vi "Tektronix_CollectWvfrm.vi"() -> ()   [LabVIEW 2018]
panel:
  in  "Collect Data":bool
  out "concatenated string":string
  out "Acquire Parameters":string
  out "output waveform 2":waveform(dbl)(graph)
  out "error out 2":errorcluster
  in  "End Point":i32
  in  "Start Point":i32
  in  "error in (no error)":errorcluster
  in  "Tektronix (0::20:)":refnum<visa-resource-name>
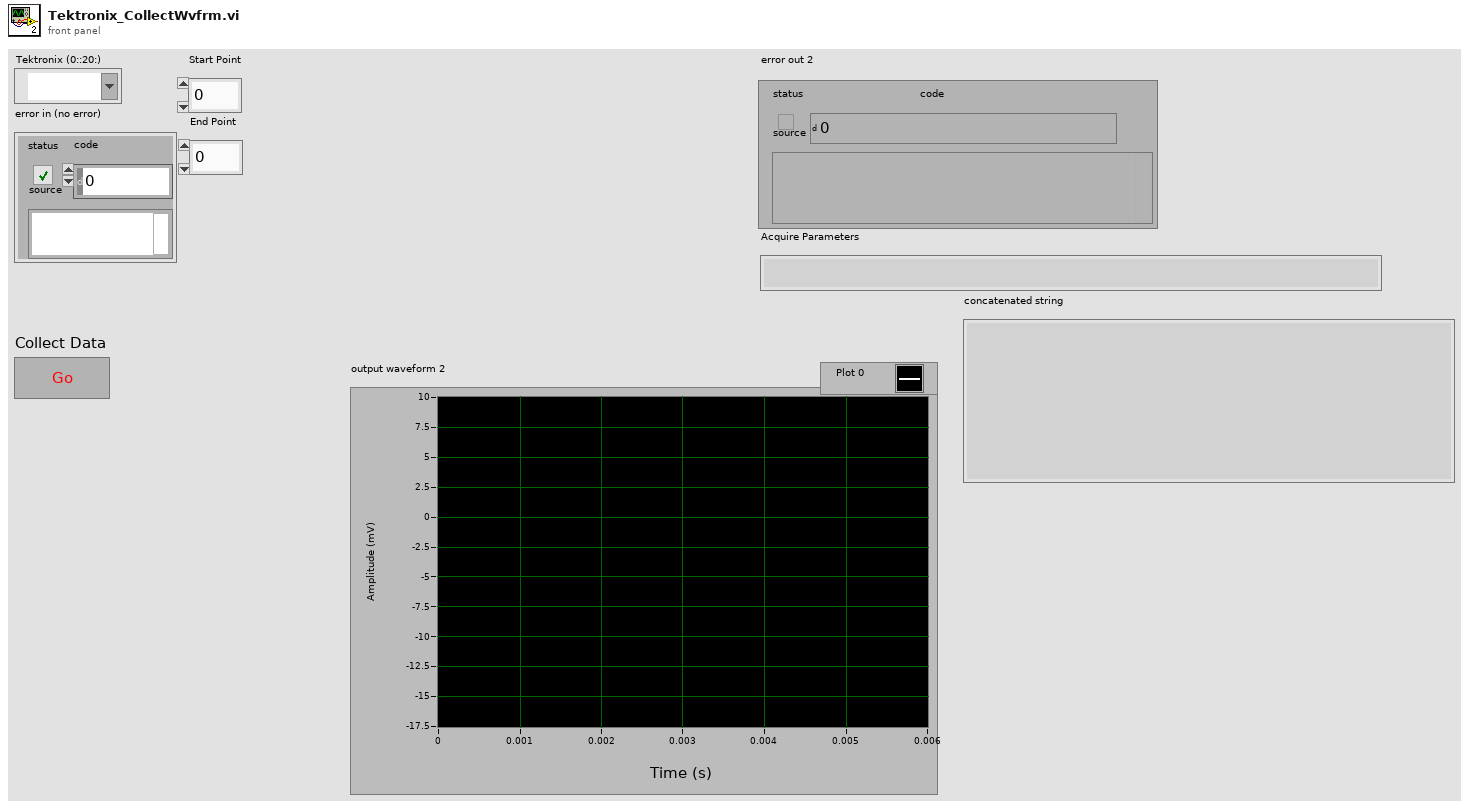
[diagram p1: front panel]
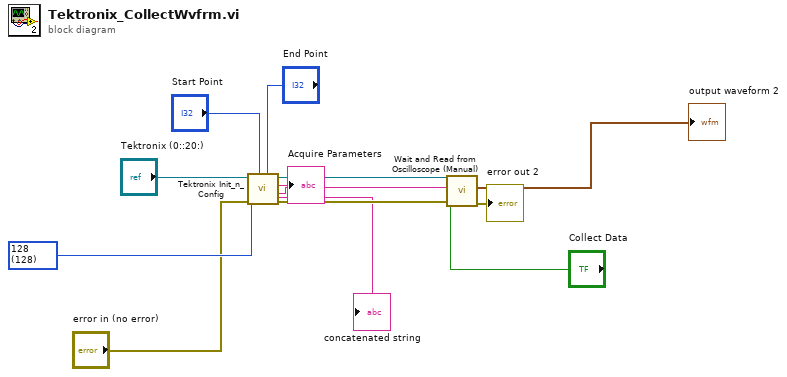
[diagram p0: block diagram]
diagram:
  w12 = u8 128 items=["128"=128, "64"=64, "16"=16, "4"=4] ("# Average")
  n1 = call "Tektronix Init_n_Config.vi"("End Point"="End Point", "Start Point"="Start Point", "error in (no error)"="error in (no error)", "# Average"=w12, "Tektronix (0::20:)"="Tektronix (0::20:)") -> ("error out"=w6:errorcluster, "Waveform Parameters"=w7:string, "Acquire Parameters"=→"Acquire Parameters":string, "VISA resource name out"=w8:refnum<visa-resource-name>, "concatenated string"=→"concatenated string":string)  [unwired: 2 in]
  n2 = call "Wait and Read from Oscilloscope (Manual).vi"("error in (no error)"=w6, "Collect Data"="Collect Data", "data format"=w7, "VISA resource name"=w8) -> ("error out 2"=→"error out 2":errorcluster, "output waveform 2"=→"output waveform 2":waveform(dbl))  [unwired: 5 in, 1 out]
